vi "PH_PPPA_PowerUnit.set safe state.vi"(0 "i ref in":refnum<vi>, 5 "error in (no error)":errorcluster) -> (14 "i ref out":refnum<vi>, 19 "error out":errorcluster)   [LabVIEW 2014, in "PH_PPPA_PowerUnit.lvlib"]
doc: "This VI set \"inistate SM\", set GUI element \"PU on\" = false, unregister PSU Info Tags, set GUI elements \"PSU Info\" = 0, set attribute \"PU on\" = false"
uses:
  PH_PPPA_PowerUnit.lvlib
  PH_Basics/PH_PowerUnit_BaseClass/PH_PowerUnit_BaseClass.lvlib
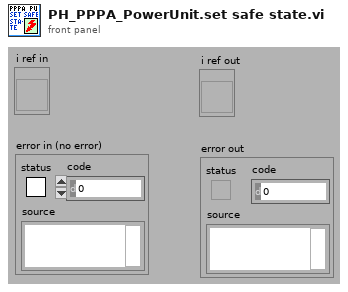
[diagram p1: front panel]
types:
  T1 = typedef "PH_PPPA_PowerUnit.lvlib/PH_PPPA_PowerUnit.i attribute.ctl" = cluster{"GUI Refs":cluster{"Ignitron":refnum<vi>, "Rossrelais":refnum<vi>, "Set Voltage":refnum<vi>, "PSU":refnum<vi>, "EOC":refnum<vi>, "Trigger":refnum<vi>}, "Ignitron":T2, "PSU":T4, "Dump Ross Relais":T5, "Trigger":cluster{"State Device":T3, "linked?":bool}, "Timing Settings":cluster{"Prdc Fast?":bool, "Default Value Periodic Interval":i32, "Mercury on since":dbl, "Warm up Time Mercury [s]":dbl}, "Set Voltage [V]":dbl, "19er Ignitionbox":string}
  T2 = typedef "PH_PP_Common.lvlib/PH_PP_Common.Ignitron Attributes.ctl" = cluster{"State Device":T3, "linked?":bool}
  T3 = typedef "PH_StatusHandler.lvlib/PH_StatusHandler.Status.ctl" = i16
  T4 = typedef "PH_PP_Common.lvlib/PH_PP_Common.PSU Attributes.ctl" = cluster{"lower limit [V]":dbl, "upper limit [V]":dbl, "Voltage set":bool, "State Device":T3, "linked?":bool}
  T5 = typedef "PH_PP_Common.lvlib/PH_PP_Common.Ross Relais Attributes.ctl" = cluster{"State Device":T3, "linked?":bool}
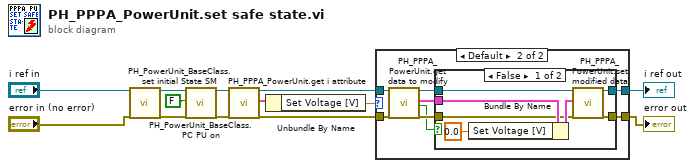
[diagram p0: block diagram]
diagram:
  n1 = call "PH_PowerUnit_BaseClass.set initial State SM.vi"("VI in"="i ref in", "error in (no error)"="error in (no error)") -> ("VI out"=w9:refnum<vi>, "error out"=w10:errorcluster)  [unwired: 16 in]
  n2 = call "PH_PowerUnit_BaseClass.PC PU on.vi"("i ref in"=w9, "PU on"=FALSE, "error in (no error)"=w10) -> ("i ref out"=w4:refnum<vi>, "error out"=w6:errorcluster)  [unwired: 15 in]
  n3 = call "PH_PPPA_PowerUnit.get i attribute.vi"("i ref in"=w4, "error in (no error)"=w6) -> ("i ref out"=w3:refnum<vi>, "i attribute"=w2:T1, "error out"=w5:errorcluster)  [unwired: 15 in]
  n4 = Unbundle By Name(w2) -> ("Set Voltage [V]"=w1:dbl)
  n5 = case shown="Default" w1 {
    tunnel: [w14 w22] -> w13
    tunnel: [w15 w20] -> w12
    tunnel: w5 -> [w14 w17]
    tunnel: w3 -> [w15 w16]
    frame 0 {
    }
    frame Default {
      n6 = call "PH_PPPA_PowerUnit.get data to modify.vi"("i ref in"=w16, "error in (no error)"=w17) -> ("i ref out"=w19:refnum<vi>, "i attribute"=w23:T1, "timed out"=w18:bool, "error out"=w21:errorcluster)  [unwired: 14 in]
      n7 = case shown="False" w18 {
        tunnel: w23 -> [w29 _]
        tunnel: [w28 w31] -> w22
        tunnel: w21 -> [w27 w31]
        tunnel: [w26 w32] -> w20
        tunnel: w19 -> [w25 w32]
        frame False {
          n8 = Bundle By Name(cluster=w29, "Set Voltage [V]"=0.0) -> (w30:T1)
          n9 = call "PH_PPPA_PowerUnit.set modified data.vi"("i ref in"=w25, "i attribute"=w30, "error in (no error)"=w27) -> ("i ref out"=w26:refnum<vi>, "error out"=w28:errorcluster)  [unwired: 15 in]
        }
        frame True {
        }
      }
    }
  }
  "error out" <- w13
  "i ref out" <- w12
